vi "FPGA Debounce Digital.vi"(0 "Input Signal":bool, 1 "Cycles to Filter":u16=5) -> (2 "Output Filtered Signal":bool)   [LabVIEW 2015]
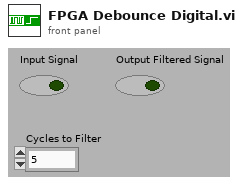
[diagram p1: front panel]
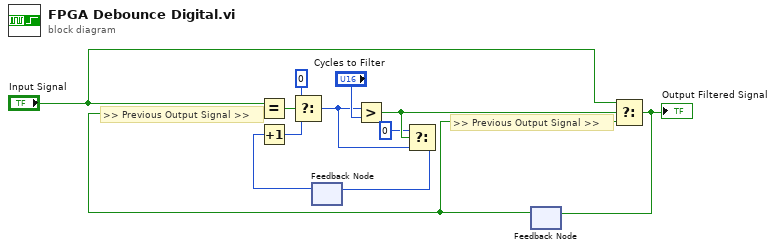
[diagram p0: block diagram]
diagram:
  # ">> Previous Output Signal >>"
  # ">> Previous Output Signal >>"
  n1 = feedback #1() -> (w11:u16)  [unwired: 1 out]
  n2 = Increment(x=w11) -> (x+1=w5:u16)
  n3 = feedback #2() -> (w7:bool)  [unwired: 1 out]
  n4 = Equal?(x="Input Signal", y=w7) -> (x = y?=w8:bool)
  n5 = Select(t=u16 0 ("f"), s=w8, f=w5) -> (s? t:f=w2:u16)
  n6 = Greater?(x=w2, y="Cycles to Filter") -> (0:w4:bool)
  n7 = Select(t=u16 0, s=w4, f=w2) -> (s? t:f=w3:u16)
  n8 = feedback-in #1(w3) -> ()
  n9 = Select(t="Input Signal", s=w4, f=w7) -> (s? t:f=w12:bool)
  "Output Filtered Signal" <- w12
  n10 = feedback-in #2(w12) -> ()
